vi "_Destroy.vi"(8 "error in (no error)":errorcluster, 11 "Minus in":refnum<class "Minus.lvclass">) -> (0 "error out":errorcluster)   [LabVIEW 2012, in "Minus.lvclass"]
uses:
  Minus.lvclass
  Readable/Readable.lvclass
  Minus.lvclass/Minus.ctl
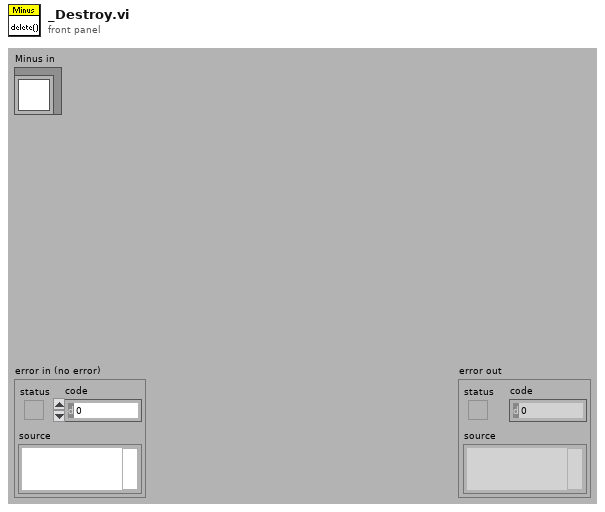
[diagram p1: front panel]
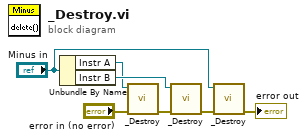
[diagram p0: block diagram]
diagram:
  n1 = Unbundle By Name("Minus in") -> ("Instr A"=w4:refnum<class "Readable.lvclass">, "Instr B"=w5:refnum<class "Readable.lvclass">)
  n2 = call-dynamic "_Destroy.vi"("error in (no error)"="error in (no error)", "Instrument in"=w4) -> ("error out"=w2:errorcluster)  [unwired: 9 out]
  n3 = call-dynamic "_Destroy.vi"("error in (no error)"=w2, "Instrument in"=w5) -> ("error out"=w1:errorcluster)  [unwired: 9 out]
  n4 = call-parent "_Destroy.vi"("error in (no error)"=w1, "Instrument in"="Minus in") -> ("error out"=→"error out":errorcluster)  [unwired: 9 out]
